vi "GetAlazar_SynthFocus_25 - ATS-SDK.vi"(1 "Digitizer Settings":T4={"Digitizer delay (us) "=0.0, "rf points per line"=2048, "lines per plane"=128, "Samp Rate (Hz)"=100000000.0, "Additional dig delay (us)"=0.0, "Voltage Scale"=0.4, "Pre-Looks"=0, "Offset delay (us)"=0.0, "bits A/D"=8, "Avg Num"=1, "DigTimeOut"=5.0, "Rel Dig Delay"=0.0, "Dig Ch"=0, "LeCroyCluster"={"LeCroy Channels"=[TRUE, FALSE, FALSE, FALSE], "LC read pt offset"=0.0, "Sweep Avg"=FALSE}, "Main Digitizer"=enum."NI Digitizer", "Dig Config"=enum."Single channel", "Digitizer ID Cluster"={"Acqiris/Alazar/SP ID"=[], "NI Instr Handles"=[], "LeCroy VISA"="", "GaGe Handle"={"Handle"=0, "Sample size"=0, "Resolution"=0, "Offset"=0, "Channels"=0, "Boards"=0}, "ATS Ref"="ATS9350", "Acqiris Address"=["PCI::INSTR0"], "ADQRef"=refnum, "adq_cu_ptr"=refnum}, "Trigger Settings"={"Trig Source"=1, "Trig Coupling"=0, "Trig Slope"=0, "Level (mV)"=1500.0}, "Bulk Acq"=FALSE, "Bulk Start Indexes"=[], "Data Ref RF"=refnum, "NI ID/Channel"=[], "Total Dig CH"=1, "Xtra Ann Trig delay (us)"=10.0, "Fix Z Delay?"=FALSE, "One Way Transmission?"=FALSE, "Data Ref Log"=refnum} {"Trigger Settings"."Trig Slope" items=["Positive", "Negative"]; "Trigger Settings"."Level (mV)" format="%.2f"; "Trigger Settings"."Trig Coupling" items=["DC 1 MOhm", "AC 1 MOhm", "DC 50 Ohm", "AC 50 Ohm"]; "Trigger Settings"."Trig Source" items=["Chan 1", "External"]; "Rel Dig Delay" format="%.2f"; "DigTimeOut" format="%.2f"; "Avg Num" min=1; "Offset delay (us)" format="%.2f"; "Additional dig delay (us)" format="%.2f"; "Digitizer delay (us)" format="%.2f"}, 2 "AlazarCluster":T8, 5 "errorin":errorcluster, 6 "File Array":string[](array[string]), 7 "Ann Array Params":T1={"Synth Foc?"=FALSE, "Focal Zones"=41, "Switch T/R"=0, "Trans Geometry (mm)"={"Transducer"=0, "Geo Focus"=12.0, "a (radius)"=3.0, "# of rings"=5, "kerf space "=0.1, "Center Freq"=12.0}, "Sub Ap Excite?"=FALSE, "Full Array Scan?"=FALSE, "Xmt/Rcv"={"XMIT"=[TRUE, TRUE, TRUE, TRUE, TRUE], "RCV"=[TRUE, TRUE, TRUE, TRUE, TRUE]}, "PulseSpacing (us)"=0.0, "Xmit Ring"=0, "XMIT CHS"=0, "RCV CHS"=0, "GPU?"=FALSE, "Save TIFF?"=FALSE, "downfactor"=1, "RCV 1CH"=0} {"RCV 1CH" items=["All", "1", "2", "3", "4", "5"]; "Trans Geometry (mm)"."Transducer" items=["6D 12R 40 MHz"=0, "10D 31R 20 MHz"=1, "10D 23R 20 MHz"=2, "6D 23R 40 MHz"=3, "4.5D 10.7R 40 MHz"=4, "9D 23.5R 20 MHz"=5, "9D 25.8R 20MHz"=6, "Enter"=99]; "Switch T/R" min=1 max=5 step=1}, 8 "lines per plane":i32, 11 "Reverse?":bool) -> (12 "Gain Array":T9(array[cluster]), 13 "Raw VGain (scale)":dbl, 15 "VGain (dB)":dbl, 19 "error out":errorcluster)   [LabVIEW 2022 SP3]
uses:
  -DigitizerRoutines/DigitizerSettings.ctl
  -DigitizerRoutines/Digitizer.ctl
  -DigitizerRoutines/DigConfig.ctl
  -DigitizerRoutines/DigitizerID.ctl
  C:/Windows/System32/ADQAPI_dotNet_helper.dll
  Annular Array/-AnnularRoutines/AnnularArray.ctl
  Annular Array/-AnnularRoutines/TransGeometry.ctl
  Annular Array/-AnnularRoutines/ArrayGeometry.ctl
  Motion Controllers/-MotionRoutines/MotionGlobals.vi
  Annular Array/-SynthApperture/ProcImageHD_I16.vi
panel:
  out "read time":u32
  out "save time":u32
  out "Numeric":i32
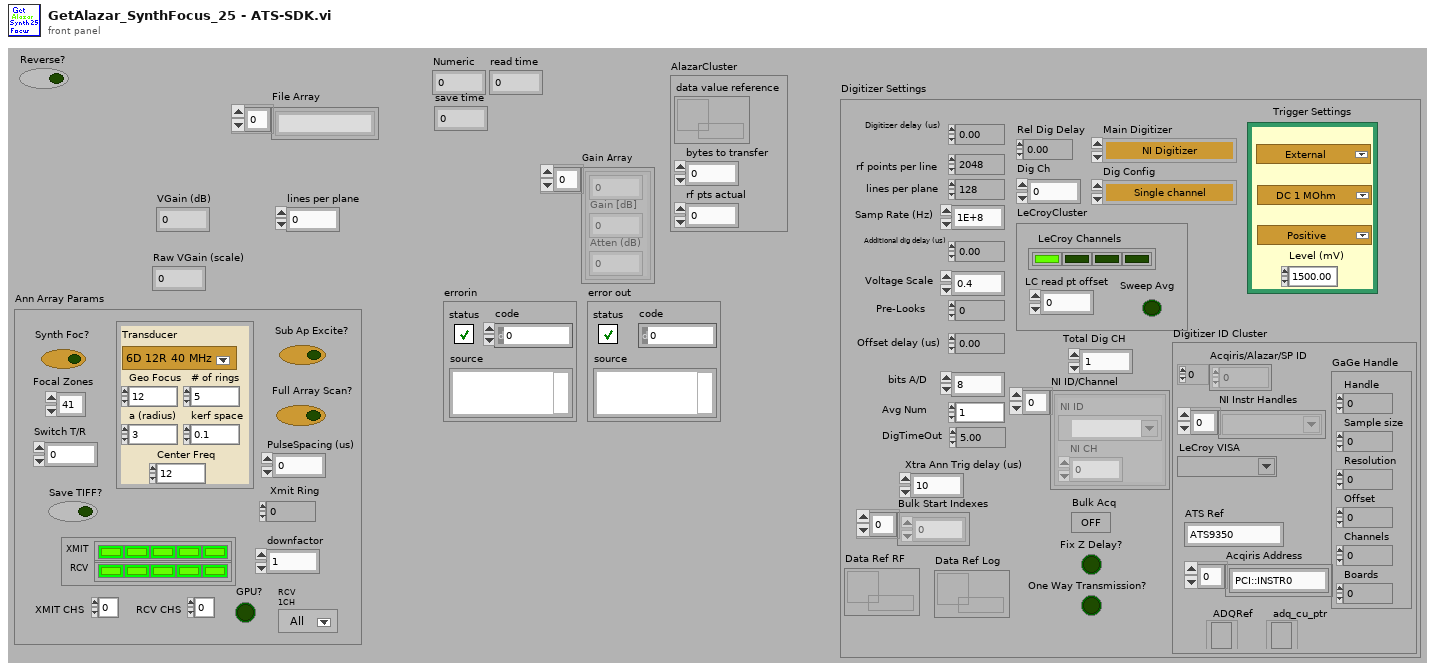
[diagram p1: front panel]
types:
  T1 = typedef "AnnularArray.ctl" = cluster{"Synth Foc?":bool, "Focal Zones":i16, "Switch T/R":i16, "Trans Geometry (mm)":T2, "Sub Ap Excite?":bool, "Full Array Scan?":bool, "Xmt/Rcv":cluster{"XMIT":bool[], "RCV":bool[]}, "PulseSpacing (us)":sgl, "Xmit Ring":i32, "XMIT CHS":u8, "RCV CHS":u8, "GPU?":bool, "Save TIFF?":bool, "downfactor":i32, "RCV 1CH":u16}
  T2 = typedef "TransGeometry.ctl" = cluster{"Transducer":T3, "Geo Focus":dbl, "a (radius)":dbl, "# of rings":i32, "kerf space ":dbl, "Center Freq":dbl}
  T3 = typedef "ArrayGeometry.ctl" = u16
  T4 = typedef "DigitizerSettings.ctl" = cluster{"Digitizer delay (us) ":dbl, "rf points per line":i32, "lines per plane":i32, "Samp Rate (Hz)":dbl, "Additional dig delay (us)":dbl, "Voltage Scale":dbl, "Pre-Looks":i32, "Offset delay (us)":dbl, "bits A/D":i8, "Avg Num":i32, "DigTimeOut":sgl, "Rel Dig Delay":sgl, "Dig Ch":i32, "LeCroyCluster":cluster{"LeCroy Channels":bool[], "LC read pt offset":dbl, "Sweep Avg":bool}, "Main Digitizer":T5, "Dig Config":T6, "Digitizer ID Cluster":T7, "Trigger Settings":cluster{"Trig Source":u16, "Trig Coupling":u16, "Trig Slope":u16, "Level (mV)":dbl}, "Bulk Acq":bool, "Bulk Start Indexes":i32[], "Data Ref RF":refnum<data-value>, "NI ID/Channel":cluster{"NI ID":refnum<k15>, "NI CH":i32}[], "Total Dig CH":i32, "Xtra Ann Trig delay (us)":dbl, "Fix Z Delay?":bool, "One Way Transmission?":bool, "Data Ref Log":refnum<data-value>}
  T5 = typedef "Digitizer.ctl" = enum16{"Acqiris Digitizer", "NI Digitizer", "LeCroy", "GaGe", "AlazarTech", "No Digitizer", "Teledyne"}
  T6 = typedef "DigConfig.ctl" = enum16{"Single channel", "2 Chans w/ 2 Acqiris", "2 Chans w/ 1 Acqiris", "5-CH Pulser New", "5-CH pulser w/ ann array", "5-pass style ann array", "Empty"}
  T7 = typedef "DigitizerID.ctl" = cluster{"Acqiris/Alazar/SP ID":u32[], "NI Instr Handles":refnum<k15>[], "LeCroy VISA":refnum<visa-resource-name>, "GaGe Handle":cluster{"Handle":u32, "Sample size":u32, "Resolution":i32, "Offset":i32, "Channels":u32, "Boards":u32}, "ATS Ref":string, "Acqiris Address":string[], "ADQRef":refnum<k24>, "adq_cu_ptr":refnum<k24>}
  T8 = cluster{"data value reference":refnum<data-value>, "bytes to transfer":u32, "rf pts actual":u32}
  T9 = cluster{sgl, "Gain [dB]  ":sgl, "Atten (dB)":sgl}[]
  T10 = cluster{"wfm":i16[][], "max queue size (-1, unlimited)":i32}
  T11 = cluster{sgl, "Gain [dB]  ":sgl, "Atten (dB)":sgl}
  T12 = cluster{"low cutoff":i32, "order":i32, "high cutoff":i32}
  T13 = cluster{"FIR Windowed Coefficients":dbl[], "Filter Prams":cluster{"low cutoff":i32, "order":i32, "high cutoff":i32}}
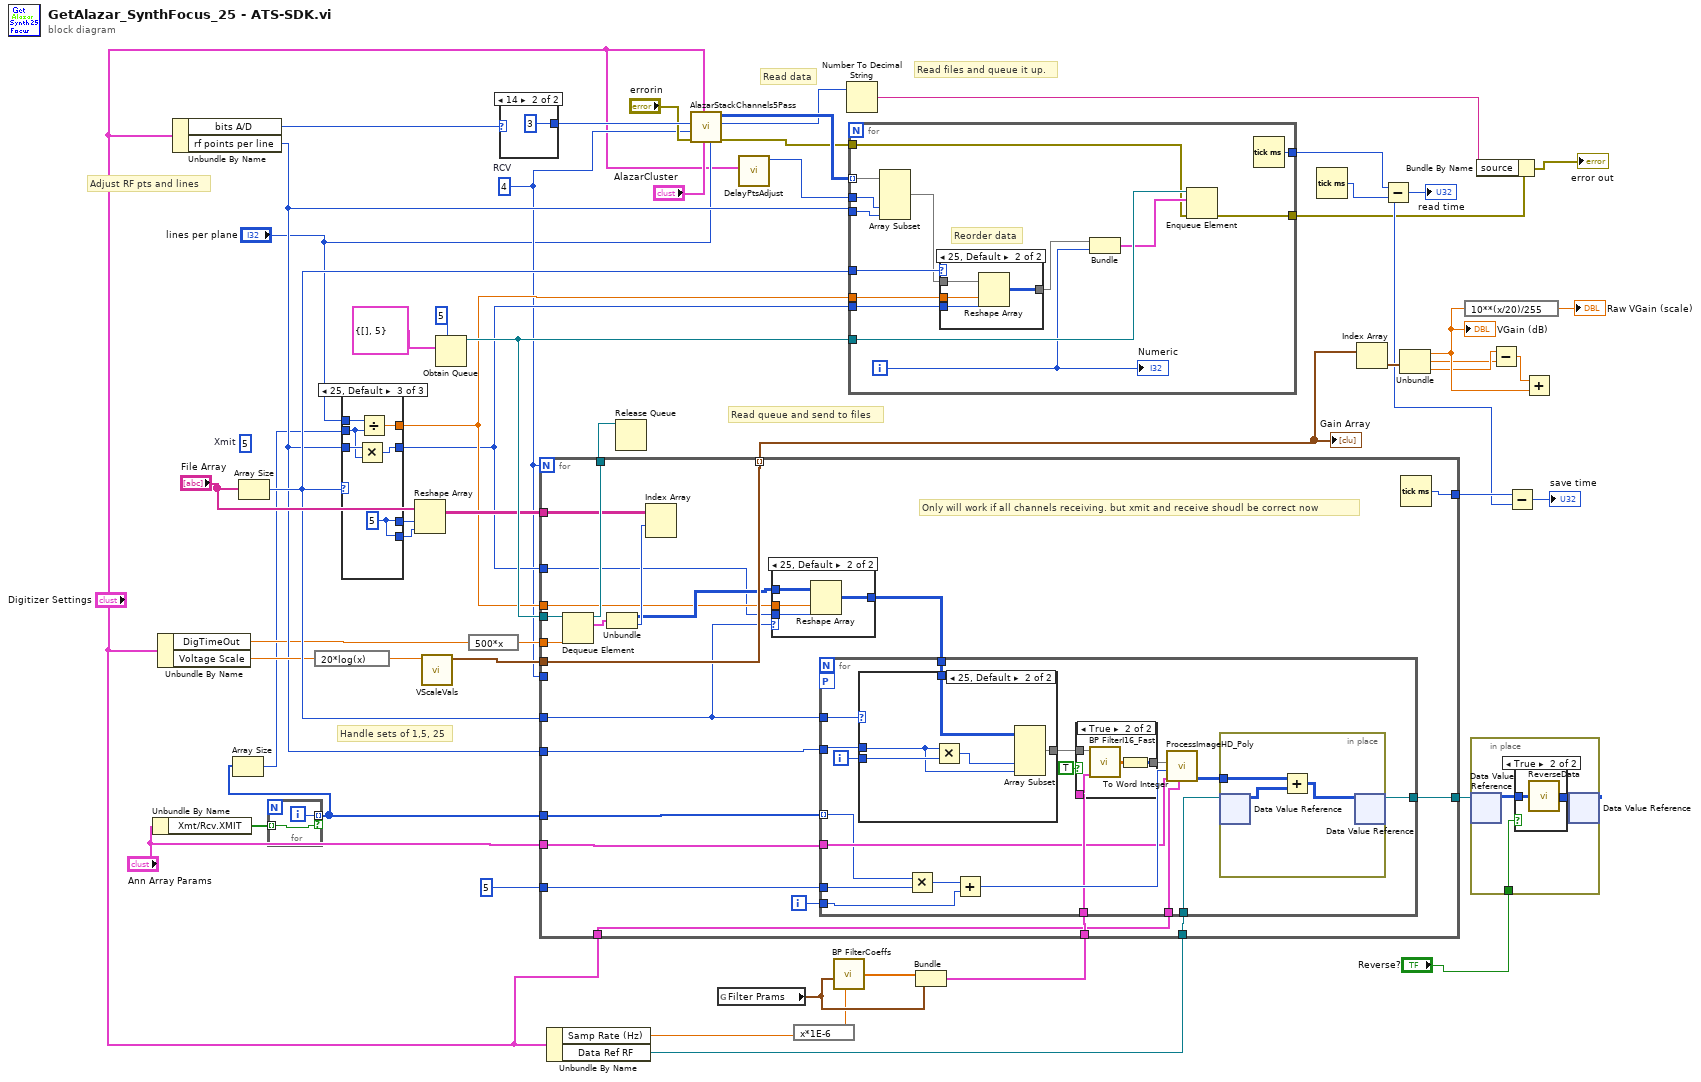
[diagram p0: block diagram]
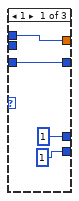
[diagram p5: hidden frame]
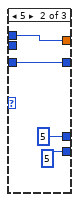
[diagram p6: hidden frame]
diagram:
  (unwired) 5  # Xmit
  w10 = 4  # RCV
  # "Read data"
  # "Adjust RF pts and lines"
  # "Handle sets of 1,5, 25"
  # "Read files and queue it up."
  # "Read queue and send to files"
  n1 = Unbundle By Name("Ann Array Params") -> ("Xmt/Rcv.XMIT"=w3:bool[])
  n2 = Unbundle By Name("Digitizer Settings") -> ("DigTimeOut"=w8:sgl, "Voltage Scale"=w23:dbl)
  n3 = Unbundle By Name("Digitizer Settings") -> ("bits A/D"=w20:i8, "rf points per line"=w21:i32)
  n4 = Array Size(array="File Array") -> (size(s)=w36:i32)
  n5 = for {
    tunnel: w3 -> [w57] mode=indexing
    tunnel: [w58] -> w2 mode=indexing if=w57
    i -> [w58]
  }
  n6 = Array Size(array=w2) -> (size(s)=w1:i32)
  n7 = expression code="20*log(x)"(w23) -> (w34:dbl)
  n8 = case shown="25, Default" w36 {
    tunnel: [1 5 w72] -> w39
    tunnel: [w61 w65 w68] -> w28
    tunnel: w21 -> [w61 w65 w69]
    tunnel: [w60 w64 w70] -> w29
    tunnel: "lines per plane" -> [w60 w64 w71]
    tunnel: [1 5 w72] -> w38
    tunnel: w1 -> [_ _ w67]
    frame 1 {
    }
    frame 5 {
    }
    frame 25, Default {
      w72 = 5
      n9 = Multiply(x=w69, y=w67) -> (x*y=w68:i32)
      n10 = Divide(x=w71, y=w67) -> (x/y=w70:dbl)
    }
  }
  n11 = Reshape Array("File Array", w39, w38) -> (w35:string[][])
  n12 = call "VScaleVals.vi"("Full Scale"=w34) -> ("Voltage Scale"=w33:T11)  [unwired: 8 in, 2 out]
  n13 = Obtain Queue(max queue size (-1, unlimited)=5, element data type=T10 {"wfm"=[], "max queue size (-1, unlimited)"=5}) -> (queue out=w48:refnum<queue>)  [unwired: 3 in, 2 out]
  n14 = expression code="500*x"(w8) -> (w37:sgl)
  n15 = case shown="14" w20 {
    tunnel: [_ u16 3 ("Extra Shift")] -> w15
    frame 0, Default {
    }
    frame 14 {
    }
  }
  n16 = Unbundle By Name("Digitizer Settings") -> ("Samp Rate (Hz)"=w22:dbl, "Data Ref RF"=w19:refnum<data-value>)
  n17 = call "AlazarStackChannels5Pass.vi"("lines per plane"="lines per plane", "AlazarCluster"="AlazarCluster", "Digitizer Settings"="Digitizer Settings", "error in"="errorin", "Channels"=w10, "Extra Shift"=w15) -> ("error out"=w12:errorcluster, "Return Code"=w13:u32, "ChStackDataOut"=w14:i16[][][])  [unwired: 2 in, 1 out]
  n18 = global read "MotionGlobals.vi" "Filter Prams"() -> (w27:T12)
  n19 = call "DelayPtsAdjust.vi"("Digitizer Settings"="Digitizer Settings") -> ("PostDelayCorrection"=w6:u32)  [unwired: 9 in, 1 out]
  n20 = expression code="x*1E-6"(w22) -> (w26:dbl)
  n21 = call "BP FilterCoeffs.vi"("sample rate MHz"=w26, "Filter Prams"=w27) -> ("FIR Windowed Coefficients"=w25:dbl[])  [unwired: 4 in]
  n22 = Number To Decimal String(number=w13) -> (decimal integer string=w31:string)  [unwired: 1 in]
  n23 = for {
    tunnel: w48 -> [w87]
    tunnel: [w85] -> w46
    tunnel: [w84] -> w32
    tunnel: w36 -> [w83]
    tunnel: w29 -> [w82]
    tunnel: w28 -> [w81]
    tunnel: w14 -> [w79] mode=indexing
    tunnel: w21 -> [w78]
    tunnel: w12 -> [w75]
    tunnel: w6 -> [w74]
    i -> [w76]
    # "Reorder data"
    n24 = Array Subset(array=w79, index (col)=w74, length (col)=w78) -> (w77:i16[][])  [unwired: 2 in]
    n25 = case shown="25, Default" w83 {
      tunnel: w81 -> [_ w92]
      tunnel: w77 -> [w88 w91]
      tunnel: [w88 w90] -> w80
      tunnel: w82 -> [_ w89]
      frame 0 {
      }
      frame 25, Default {
        n26 = Reshape Array(w91, w89, w92) -> (w90:i16[][])
      }
    }
    n27 = Bundle(w80, w76) -> (w86:cluster{i16[][], i32})  [unwired: 1 in]
    n28 = Enqueue Element(queue=w87, element=w86, error in (no error)=w75) -> (error out=w84:errorcluster)  [unwired: 1 in, 2 out]
    n29 = Tick Count (ms)() -> (millisecond timer value=w85:u32)
    "Numeric" <- w76
  }
  n30 = Bundle("FIR Windowed Coefficients"=w25, "Filter Prams"=w27) -> (w24:T13)  [unwired: 1 in]
  n31 = for {
    N: w10 -> [_]
    tunnel: w21 -> [w102]
    tunnel: [w108] -> w49 mode=indexing
    tunnel: w48 -> [w114]
    tunnel: [w112] -> w41
    tunnel: [w111] -> w45
    tunnel: w36 -> [w101]
    tunnel: w37 -> [w110]
    tunnel: w35 -> [w109]
    tunnel: w33 -> [w108]
    tunnel: w29 -> [w105]
    tunnel: w28 -> [w104]
    tunnel: w24 -> [w100]
    tunnel: w19 -> [w99]
    tunnel: w10 -> [_]
    tunnel: "Digitizer Settings" -> [w97]
    tunnel: "Ann Array Params" -> [w96]
    tunnel: [w95] -> w18
    tunnel: 5 -> [w94]
    tunnel: w2 -> [w93]
    i -> [w98]
    # "Only will work if all channels receiving. but xmit and receive shoudl be correct now"
    n32 = Dequeue Element(queue=w114, timeout in ms (-1)=w110) -> (queue out=w112:refnum<queue>, element=w113:T10)  [unwired: 1 in, 2 out]
    n33 = Unbundle(w113) -> ("wfm"=w106:i16[][], "max queue size (-1, unlimited)"=w107:i32)
    n34 = Index Array(array=w109, index (row)=w107) -> ()  [unwired: 1 in, 1 out]
    n35 = case shown="25, Default" w101 {
      tunnel: w104 -> [_ w151]
      tunnel: w106 -> [w147 w150]
      tunnel: [w147 w149] -> w103
      tunnel: w105 -> [_ w148]
      frame 0 {
      }
      frame 25, Default {
        n36 = Reshape Array(w150, w148, w151) -> (w149:i16[][])
      }
    }
    n37 = for {
      tunnel: w102 -> [w132]
      tunnel: w103 -> [w131]
      workers-P: _ -> [_]
      tunnel: w101 -> [w130]
      tunnel: w99 -> [w125]
      tunnel: w100 -> [w122]
      tunnel: w98 -> [w120]
      tunnel: w97 -> [w119]
      tunnel: w96 -> [w118]
      tunnel: [w117] -> w95
      tunnel: w94 -> [w116]
      tunnel: w93 -> [w115] mode=indexing
      i -> [w129]
      n38 = case shown="25, Default" w130 {
        tunnel: [w141 w142] -> w124
        tunnel: w129 -> [_ w146]
        tunnel: w132 -> [_ w144]
        tunnel: w131 -> [w141 w143]
        frame 5 {
        }
        frame 25, Default {
          n39 = Multiply(x=w144, y=w146) -> (x*y=w145:i32)
          n40 = Array Subset(array=w143, index (col)=w145, length (col)=w144) -> (w142:i16[][])  [unwired: 2 in]
        }
      }
      n41 = Multiply(x=w115, y=w116) -> (x*y=w128:i32)
      n42 = Add(x=w128, y=w120) -> (x+y=w127:i32)
      n43 = case shown="True" TRUE {
        tunnel: w124 -> [w133 w136]
        tunnel: [w133 w135] -> w123
        tunnel: w122 -> [_ w134]
        frame False {
        }
        frame True {
          n44 = call "BP FilterI16_Fast.vi"("Filter"=w134, "Array in"=w136) -> ("Filtered X"=w137:dbl[][])  [unwired: 4 in]
          n45 = To Word Integer(number=w137) -> (16bit integer=w135:i16[][])
        }
      }
      n46 = call-poly "ProcessImageHD_Poly.vi"("Digitizer Settings"=w119, "Ann Array Params"=w118, "T/R Ring"=w127, "Scan Data In"=w123) -> ("Synth App Out"=w126:i16[][])  [unwired: 4 in, 1 out]
      n47 = in-place {
        in-place-border: w126 -> [w138]
        n48 = in-place-dvr #1(w125) -> (w140:i16[][])  [unwired: 1 out]
        n49 = Add(x=w138, y=w140) -> (x+y=w139:i16[][])
        n50 = in-place-dvr #1(w139) -> (w117:refnum<data-value>)  [unwired: 1 out]
      }
    }
    n51 = Tick Count (ms)() -> (millisecond timer value=w111:u32)
  }
  "Gain Array" <- w49
  n52 = Release Queue(queue=w41) -> ()  [unwired: 2 in, 3 out]
  n53 = Tick Count (ms)() -> (millisecond timer value=w44:u32)
  n54 = Index Array(array=w49) -> (element=w56:T11)  [unwired: 1 in]
  n55 = Subtract(x=w46, y=w44) -> (x-y=→"read time":u32)
  n56 = Unbundle(w56) -> (w55:sgl, "Gain [dB]"=w53:sgl, "Atten (dB)"=w54:sgl)
  "VGain (dB)" <- w55
  n57 = expression code="10**(x/20)/255"(w55) -> (→"Raw VGain (scale)":sgl)
  n58 = in-place {
    in-place-border: "Reverse?" -> [w152]
    n59 = in-place-dvr #2(w18) -> (w154:i16[][])  [unwired: 1 out]
    n60 = case shown="True" w152 {
      tunnel: w154 -> [w155 w157]
      tunnel: [w155 w156] -> w153
      frame False {
      }
      frame True {
        n61 = call "ReverseData.vi"("Array in"=w157) -> ("Array out"=w156:i16[][])
      }
    }
    n62 = in-place-dvr #2(w153) -> ()  [unwired: 2 out]
  }
  n63 = Bundle By Name(cluster=w32, "source"=w31) -> (→"error out":errorcluster)
  n64 = Subtract(x=w54, y=w53) -> (x-y=w52:sgl)
  n65 = Subtract(x=w45, y=w44) -> (x-y=→"save time":u32)
  n66 = Add(x=w52, y=w55) -> ()  [unwired: 1 out]
